vi "Launch Pane Relief Tool For Example Panel.vi"   [LabVIEW 2015]
panel:
  # "RUN THIS VI TO TEST THE PANE RELIEF TOOL"
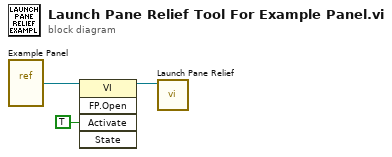
[diagram p0: block diagram]
diagram:
  n1 = vi-ref "Example Panel.vi"() -> (w3:refnum<vi>)
  n2 = invoke class="VI" method="FP.Open"(reference=w3, "Activate"=TRUE ("Activate?")) -> (reference out=w1:refnum<vi>)  [unwired: 3 in, 4 out]
  n3 = call "Launch Pane Relief.vi"("VI in"=w1) -> ()  [unwired: 9 in, 2 out]
